vi "auto_alignment-make_start_simplex.vi"(8 "L":dbl=1.0 format="%#_13g", 10 "yStart":dbl, 11 "xStart":dbl) -> (3 "Array":dbl[][](array[numeric]))   [LabVIEW 2024]
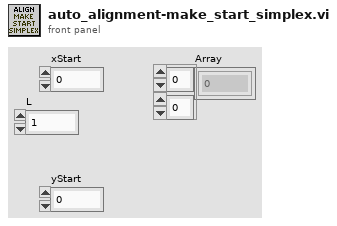
[diagram p1: front panel]
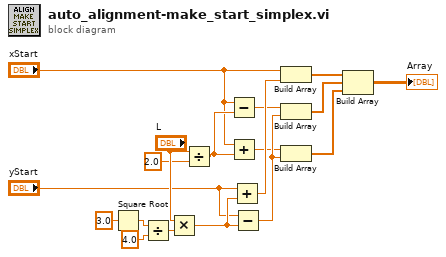
[diagram p0: block diagram]
diagram:
  n1 = Square Root(x=3.0) -> (sqrt(x)=w5:dbl)
  n2 = Divide(x=w5, y=4.0) -> (x/y=w16:dbl)
  n3 = Multiply(x="L", y=w16) -> (x*y=w17:dbl)
  n4 = Divide(x="L", y=2.0) -> (x/y=w15:dbl)
  n5 = Subtract(x="xStart", y=w15) -> (x-y=w8:dbl)
  n6 = Add(x="xStart", y=w15) -> (x+y=w9:dbl)
  n7 = Add(x="yStart", y=w17) -> (x+y=w10:dbl)
  n8 = Subtract(x="yStart", y=w17) -> (x-y=w11:dbl)
  n9 = Build Array("xStart", w10) -> (w4:dbl[])
  n10 = Build Array(w8, w11) -> (w3:dbl[])
  n11 = Build Array(w9, w11) -> (w2:dbl[])
  n12 = Build Array(w4, w3, w2) -> (→"Array":dbl[][])
